vi "test-ControllerUtil-manual-entry.vi"() -> (3 "All Tests Passed":bool)   [LabVIEW 2019]
uses:
  <vilib>/Rock Robotics/WPI/ThirdParty/JAS_Junk/TrajLib/Trajectory_Library.lvlib
panel:
  out "T1  = -20":dbl
  out "T0  = -20":dbl
  in  "Maximum_Input":dbl
  in  "Minimum_Input":dbl
  in  "Measurerment(PV)":dbl step=10.0
  in  "Reference(SP)":dbl step=10.0
  out "Error":dbl
  # "Controller Util -- Modulus Error test..."
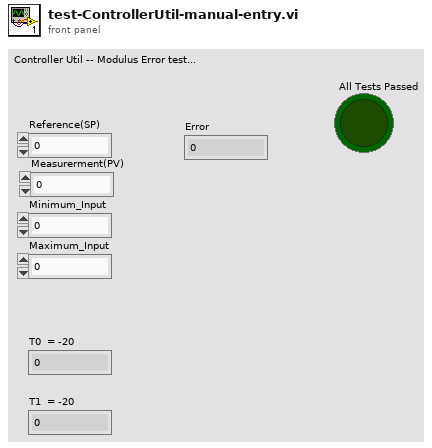
[diagram p1: front panel]
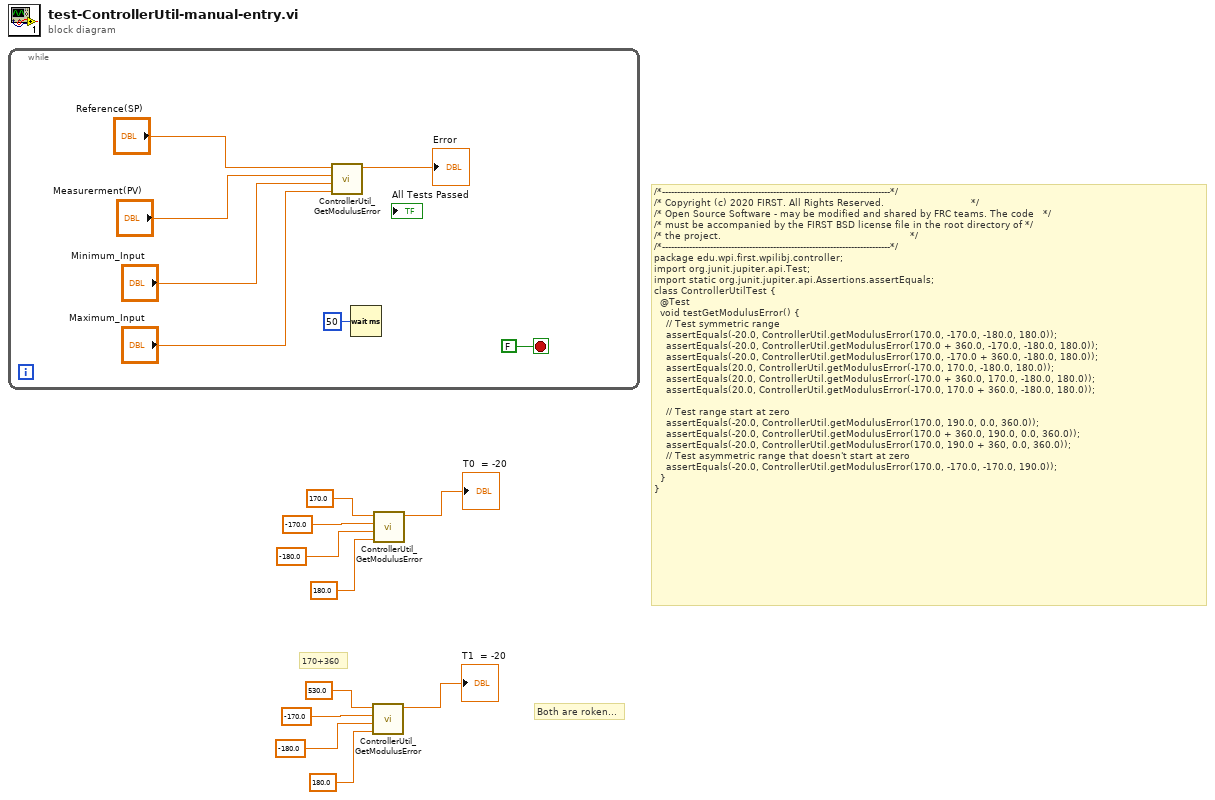
[diagram p0: block diagram]
diagram:
  # "Both are roken..."
  # "170+360"
  # "/*----------------------------------------------------------------------------*/\n/* Copyright (c) 2020 FIRST. All Rights Reserved.                             */\n/* Open Source Software - may be modified and shared by FRC teams. The code   */\n/* must be accompanied by the FIRST BSD license file in the root directory of */\n/* the project.                                                               */\n/*----------------------------------------------------------------------------*/\npackage edu.wpi.first.wpilibj.controller;\nimport org.junit.jupiter.api.Test;\nimport static org.junit.jupiter.api.Assertions.assertEquals;\nclass ControllerUtilTest {\n  @Test\n  void testGetModulusError() {\n    // Test symmetric range\n    assertEquals(-20.0, ControllerUtil.getModulusError(170.0, -170.0, -180.0, 180.0));\n    assertEquals(-20.0, ControllerUtil.getModulusError(170.0 + 360.0, -170.0, -180.0, 180.0));\n    assertEquals(-20.0, ControllerUtil.getModulusError(170.0, -170.0 + 360.0, -180.0, 180.0));\n    assertEquals(20.0, ControllerUtil.getModulusError(-170.0, 170.0, -180.0, 180.0));\n    assertEquals(20.0, ControllerUtil.getModulusError(-170.0 + 360.0, 170.0, -180.0, 180.0));\n    assertEquals(20.0, ControllerUtil.getModulusError(-170.0, 170.0 + 360.0, -180.0, 180.0));\n\n    // Test range start at zero\n    assertEquals(-20.0, ControllerUtil.getModulusError(170.0, 190.0, 0.0, 360.0));\n    assertEquals(-20.0, ControllerUtil.getModulusError(170.0 + 360.0, 190.0, 0.0, 360.0));\n    assertEquals(-20.0, ControllerUtil.getModulusError(170.0, 190.0 + 360, 0.0, 360.0));\n    // Test asymmetric range that doesn't start at zero\n    assertEquals(-20.0, ControllerUtil.getModulusError(170.0, -170.0, -170.0, 190.0));\n  }\n}"
  n1 = while {
    stop <- FALSE stop-if-true
    n2 = call <vilib>:"ControllerUtil_GetModulusError.vi"("Maximum_Input"="Maximum_Input", "Minimum_Input"="Minimum_Input", "Measurerment(PV)"="Measurerment(PV)", "Reference(SP)"="Reference(SP)") -> ("Error"=→"Error":dbl)  [unwired: 7 in]
    n3 = Wait (ms)(milliseconds to wait=u32 50) -> ()  [unwired: 1 out]
  }
  n4 = call <vilib>:"ControllerUtil_GetModulusError.vi"("Maximum_Input"=180.0, "Minimum_Input"=-180.0, "Measurerment(PV)"=-170.0, "Reference(SP)"=530.0) -> ("Error"=→"T1  = -20":dbl)  [unwired: 7 in]
  n5 = call <vilib>:"ControllerUtil_GetModulusError.vi"("Maximum_Input"=180.0, "Minimum_Input"=-180.0, "Measurerment(PV)"=-170.0, "Reference(SP)"=170.0) -> ("Error"=→"T0  = -20":dbl)  [unwired: 7 in]
